vi "bypass_block.vi"(2 "Control":T3, 3 "A":T4) -> (0 "Flags":T1, 1 "Result":T2)   [LabVIEW 2013]
panel:
  # "R1"
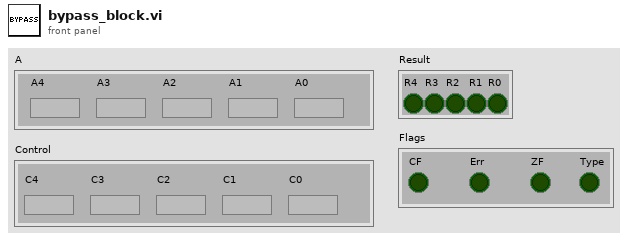
[diagram p1: front panel]
types:
  T1 = cluster{"CF":bool, "Err":bool, "ZF":bool, "Type":bool}
  T2 = cluster{"R4":bool, "R3":bool, "R2":bool, bool, "R0":bool}
  T3 = cluster{"C4":bool, "C3":bool, "C2":bool, "C1":bool, "C0":bool}
  T4 = cluster{"A4":bool, "A3":bool, "A2":bool, "A1":bool, "A0":bool}
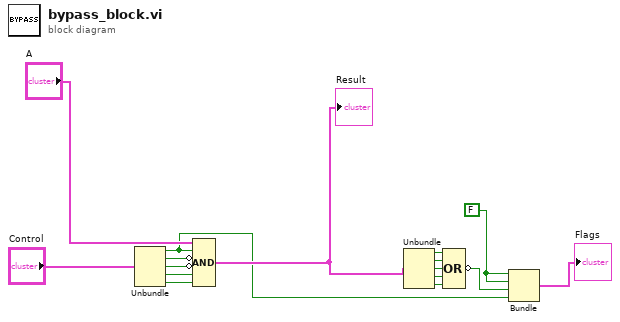
[diagram p0: block diagram]
diagram:
  w3 = FALSE
  n1 = Unbundle("Control") -> ("C4"=w1:bool, "C3"=w15:bool, "C2"=w14:bool, "C1"=w13:bool, "C0"=w12:bool)
  n2 = Compound Arithmetic op=AND("A", w1, invert w15, invert w14, w13, w12) -> (w5:T4)
  "Result" <- w5
  n3 = Unbundle(w5) -> ("A4"=w10:bool, "A3"=w9:bool, "A2"=w8:bool, "A1"=w7:bool, "A0"=w6:bool)
  n4 = Compound Arithmetic op=OR(w10, w9, w8, w7, w6) -> (invert w4:bool)
  n5 = Bundle(w3, w3, w4, "C4"=w1) -> (→"Flags":cluster{bool, bool, bool, "C4":bool})  [unwired: 1 in]
